vi "Read GPS.vi"(0 "VISA resource name":refnum<visa-resource-name>="COM1", 5 "timeout (ms)":u32=10000, 7 "UTC Time Zone":i32=-5, 9 "stop":bool, 11 "error in (no error)":errorcluster) -> (4 "GPS Data":T1 {"Course over ground (degrees)" format="%#.6g"; "Speed over ground (knots)" format="%#.6g"; "Magnetic Variation (degrees)" format="%#.6g"; "Longitude (ddmm.mmmm)" format="%#.6g"; "Lattitude (ddmm.mmmm)" format="%#.6g"}, 6 "GPS Data Valid?":bool, 10 "Stopped?":bool, 15 "error out":errorcluster)   [LabVIEW 2011]
doc: "This subVI decodes the most common NMEA-0183 sentence transmitted by GPS receivers, the $GPRMC sentence. The subvi returns time, position, ground speed, and magnetic variation. In the GPS interface configuration, use the \"NMEA OUT\" setting and set the baud rate to the standard 4800 bps setting. Connected to the computer's serial port using a PC Interface Cable, available from the GPS vendor. This subvi initializes the serial port on first call. On subsequent calls, the initialization is skipped. Always use the Stop input when stopping the VI so that the serial port connection is closed."
uses:
  <vilib>/Instr/_visa.llb/VISA Configure Serial Port (Instr).vi
panel:
  in  "Cluster":T1 {"Course over ground (degrees)" format="%_4g"; "Speed over ground (knots)" format="%_3g"; "Magnetic Variation (degrees)" format="%_4g"; "Longitude (ddmm.mmmm)" format="%_8g"; "Lattitude (ddmm.mmmm)" format="%_8g"}
  out "Variation East/West":string
  out "Magnetic Variation (degrees)":dbl format="%_4g"
  out "Course over ground (degrees)":dbl format="%_4g"
  out "Speed over ground (knots)":dbl format="%_3g"
  out "Longitude East/West":string
  out "Longitude (ddmm.mmmm)":dbl format="%_8g"
  out "Lattitude North/South":string
  out "Lattitude (ddmm.mmmm)":dbl format="%_8g"
  out "Local Time":timestamp
  out "UTC Time":timestamp
  in  "date time rec":T2
  out "Bytes read":u32
  out "String Read":string="\n"
  # "This subVI decodes the most common NMEA-0183 sentence transmitted by GPS receivers, the $GPRMC sentence. The subvi returns time, position, ground speed, and magnetic variation. In the GPS interface configuration, use the \"NMEA OUT\" setting and set the baud rate to the standard 4800 bps setting. Connected to the computer's serial port using a PC Interface Cable, available from the GPS vendor. This subvi initializes the serial port on first call. On subsequent calls, the initialization is skipped. Always use the Stop input when stopping the VI so that the serial port connection is closed."
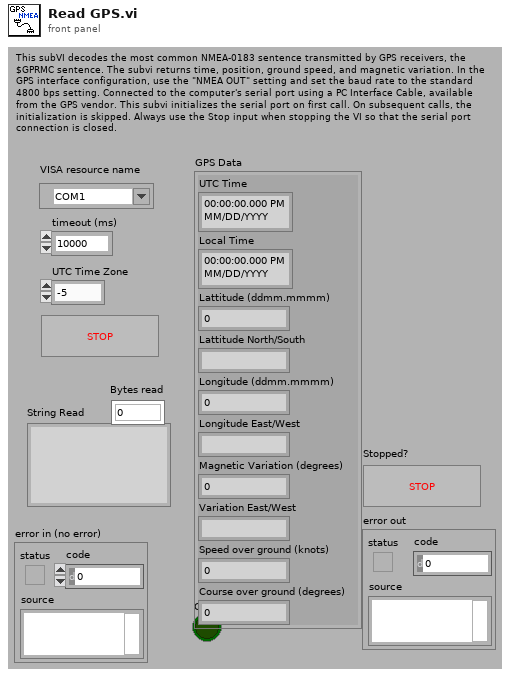
[diagram p1: front panel]
types:
  T1 = cluster{"UTC Time":timestamp, "Local Time":timestamp, "Lattitude (ddmm.mmmm)":dbl, "Lattitude North/South":string, "Longitude (ddmm.mmmm)":dbl, "Longitude East/West":string, "Magnetic Variation (degrees)":dbl, "Variation East/West":string, "Speed over ground (knots)":dbl, "Course over ground (degrees)":dbl}
  T2 = cluster{"second":i32, "minute":i32, "hour":i32, "day of month":i32, "month":i32, "year":i32, "day of week":i32, "day of year":i32, "is DST":i32}
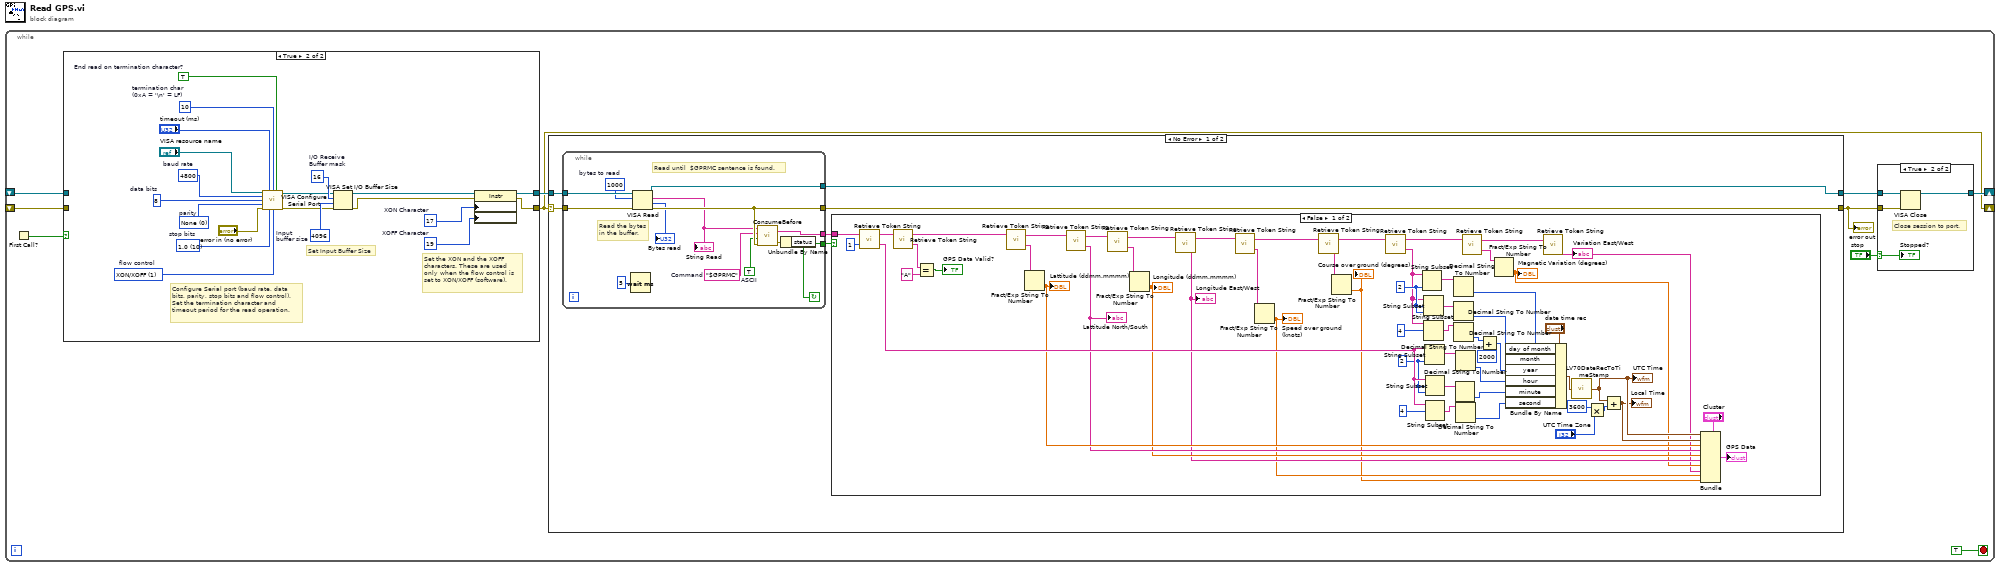
[diagram p0: block diagram]
diagram:
  n1 = while {
    shift-right: [w5] -> _
    shift-left: _ -> [w4]
    shift-right: [w3] -> _
    shift-left: _ -> [w2]
    stop <- TRUE stop-if-true
    n2 = First Call?() -> (First Call?: T/F=w8:bool)
    n3 = case shown="True" w8 {
      tunnel: [w16 w21] -> w10
      tunnel: [w15 w18] -> w3
      tunnel: w4 -> [w16 _]
      tunnel: w2 -> [w15 _]
      frame False {
      }
      frame True {
        w31 = TRUE  # End read on termination character?
        w23 = u8 19  # XOFF Character
        w24 = u8 17  # XON Character
        w29 = u32 4096  # Input buffer size
        w27 = u16 1 items=["None"=0, "XON/XOFF"=1, "RTS/CTS"=2, "DTR/DSR"=4]  # flow control
        w33 = u16 10 items=["1.0"=10, "1.5"=15, "2.0"=20]  # stop bits
        w34 = u16 0 items=["None", "Odd", "Even", "Mark", "Space"]  # parity
        w22 = u16 8  # data bits
        w36 = u32 4800  # baud rate
        w28 = u8 10  # termination char (0xA = '\n' = LF)
        w30 = u16 16  # I/O Receive Buffer mask
        # "Set the XON and the XOFF\ncharacters. These are used\nonly when the flow control is\nset to XON/XOFF (software)."
        # "Configure Serial port (baud rate, data\nbits, parity, stop bits and flow control).\nSet the termination character and\ntimeout period for the read operation."
        # "Set Input Buffer Size"
        n4 = call-poly "VISA Configure Serial Port"("VISA resource name"="VISA resource name", "timeout (10sec)"="timeout (ms)", "termination char\n(0xA = '\\n' = LF)"=w28, "Enable Termination\nChar (T)"=w31, "baud rate (9600)"=w36, "data bits (8)"=w22, "parity (0:none)"=w34, "error in (no error)"="error in (no error)", "stop bits (10: 1 bit)"=w33, "flow control (0:none)"=w27) -> ("VISA resource name out"=w20:refnum<visa-resource-name>, "error out"=w19:errorcluster)  [unwired: 4 in]
        n5 = VISA Set I/O Buffer Size(VISA resource name=w20, mask (16)=w30, size (4096)=w29, error in (no error)=w19) -> (VISA resource name out=w26:refnum<visa-resource-name>, error out=w25:errorcluster)
        n6 = property class="Instr"(reference=w26, error in=w25, "Serial Settings:Flow Control XON Character"=w24, "Serial Settings:Flow Control XOFF Character"=w23) -> (reference out=w21:refnum<visa-resource-name>, error out=w18:errorcluster)
      }
    }
    n7 = case shown="No Error" w3 {
      selector: w3 -> [w39 w113]
      tunnel: w10 -> [w42 w114]
      tunnel: [w41 w114] -> w9
      tunnel: [w40 w113] -> w1
      frame No Error {
        n8 = while {
          tunnel: w42 -> [w55]
          tunnel: [w54] -> w41
          tunnel: [w53] -> w40
          tunnel: w39 -> [w52]
          tunnel: [w48] -> w38
          tunnel: [w44] -> w37
          stop <- w44 continue-if-true
          w46 = u32 1000  # bytes to read
          w51 = "$GPRMC"  # Command
          w50 = TRUE  # ASCII
          # "Read until  $GPRMC sentence is found."
          # "Read the bytes\nin the buffer."
          n9 = Wait (ms)(milliseconds to wait=u32 5 ("millisecond multiple")) -> ()  [unwired: 1 out]
          n10 = VISA Read(VISA resource name=w55, byte count=w46, error in (no error)=w52) -> (VISA resource name out=w54:refnum<visa-resource-name>, read buffer=w49:string, return count=→"Bytes read":u32, error out=w53:errorcluster)
          "String Read" <- w49
          n11 = call <vilib>:"ConsumeBefore.vi"("error in"=w53, "ASCII"=w50, "Before"=w51, "Response String In"=w49) -> ("error out"=w47:errorcluster, "Response String Out"=w48:string)
          n12 = Unbundle By Name(w47) -> ("status"=w44:bool)
        }
        n13 = case shown="False" w37 {
          tunnel: w38 -> [w110 _]
          frame False {
            w78 = 2 ("length (rest)")
            w100 = 2 ("length (rest)")
            n14 = call "Retrieve Token String.vi"("Offset (0)"=1, "input string"=w110) -> ("token string"=w107:string, "output string"=w108:string)
            n15 = call "Retrieve Token String.vi"("input string"=w108) -> ("token string"=w112:string, "output string"=w106:string)  [unwired: 1 in]
            n16 = Equal?(x=w112, y="A") -> (x = y?=→"GPS Data Valid?":bool)
            n17 = call "Retrieve Token String.vi"("input string"=w106) -> ("token string"=w91:string, "output string"=w90:string)  [unwired: 1 in]
            n18 = Fract/Exp String To Number(string=w91) -> (number=w65:dbl)  [unwired: 3 in, 1 out]
            "Lattitude (ddmm.mmmm)" <- w65
            n19 = call "Retrieve Token String.vi"("input string"=w90) -> ("token string"=w64:string, "output string"=w89:string)  [unwired: 1 in]
            "Lattitude North/South" <- w64
            n20 = call "Retrieve Token String.vi"("input string"=w89) -> ("token string"=w88:string, "output string"=w87:string)  [unwired: 1 in]
            n21 = Fract/Exp String To Number(string=w88) -> (number=w63:dbl)  [unwired: 3 in, 1 out]
            "Longitude (ddmm.mmmm)" <- w63
            n22 = call "Retrieve Token String.vi"("input string"=w87) -> ("token string"=w62:string, "output string"=w86:string)  [unwired: 1 in]
            "Longitude East/West" <- w62
            n23 = call "Retrieve Token String.vi"("input string"=w86) -> ("token string"=w85:string, "output string"=w84:string)  [unwired: 1 in]
            n24 = Fract/Exp String To Number(string=w85) -> (number=w59:dbl)  [unwired: 3 in, 1 out]
            "Speed over ground (knots)" <- w59
            n25 = call "Retrieve Token String.vi"("input string"=w84) -> ("token string"=w83:string, "output string"=w82:string)  [unwired: 1 in]
            n26 = Fract/Exp String To Number(string=w83) -> (number=w58:dbl)  [unwired: 3 in, 1 out]
            "Course over ground (degrees)" <- w58
            n27 = call "Retrieve Token String.vi"("input string"=w82) -> ("token string"=w76:string, "output string"=w70:string)  [unwired: 1 in]
            n28 = String Subset(string=w76, length (rest)=w78) -> (substring=w77:string)  [unwired: 1 in]
            n29 = String Subset(string=w76, offset (0)=w78, length (rest)=w78) -> (substring=w79:string)
            n30 = String Subset(string=w76, offset (0)=4) -> (substring=w81:string)  [unwired: 1 in]
            n31 = String Subset(string=w107, length (rest)=w100) -> (substring=w104:string)  [unwired: 1 in]
            n32 = String Subset(string=w107, offset (0)=w100, length (rest)=w100) -> (substring=w98:string)
            n33 = String Subset(string=w107, offset (0)=4) -> (substring=w96:string)  [unwired: 1 in]
            n34 = Decimal String To Number(string=w79) -> (number=w74:i32)  [unwired: 2 in, 1 out]
            n35 = Decimal String To Number(string=w77) -> (number=w75:i32)  [unwired: 2 in, 1 out]
            n36 = Decimal String To Number(string=w81) -> (number=w73:i32)  [unwired: 2 in, 1 out]
            n37 = Decimal String To Number(string=w98) -> (number=w99:i32)  [unwired: 2 in, 1 out]
            n38 = Decimal String To Number(string=w104) -> (number=w101:i32)  [unwired: 2 in, 1 out]
            n39 = Decimal String To Number(string=w96) -> (number=w95:i32)  [unwired: 2 in, 1 out]
            n40 = call "Retrieve Token String.vi"("input string"=w70) -> ("token string"=w69:string, "output string"=w68:string)  [unwired: 1 in]
            n41 = Add(x=w73, y=2000) -> (x+y=w71:i32)
            n42 = Fract/Exp String To Number(string=w69) -> (number=w61:dbl)  [unwired: 3 in, 1 out]
            "Magnetic Variation (degrees)" <- w61
            n43 = Bundle By Name(cluster="date time rec", "day of month"=w75, "month"=w74, "year"=w71, "hour"=w101, "minute"=w99, "second"=w95) -> (w103:T2)
            n44 = call "Retrieve Token String.vi"("input string"=w68) -> ("token string"=w60:string)  [unwired: 1 in, 1 out]
            "Variation East/West" <- w60
            n45 = call <vilib>:"LV70DateRecToTimeStamp.vi"("date time rec"=w103) -> ("Time Stamp"=w67:timestamp)
            "UTC Time" <- w67
            n46 = Multiply(x=3600 ("number"), y="UTC Time Zone") -> (x*y=w92:i32)
            n47 = Add(x=w67, y=w92) -> (x+y=w66:timestamp)
            "Local Time" <- w66
            n48 = Bundle(cluster="Cluster", "UTC Time"=w67, "Local Time"=w66, "Lattitude (ddmm.mmmm)"=w65, "Lattitude North/South"=w64, "Longitude (ddmm.mmmm)"=w63, "Longitude East/West"=w62, "Magnetic Variation (degrees)"=w61, "Variation East/West"=w60, "Speed over ground (knots)"=w59, "Course over ground (degrees)"=w58) -> (→"GPS Data":T1)
          }
          frame True {
          }
        }
      }
      frame Error {
      }
    }
    "error out" <- w1
    n49 = case shown="True" "stop" {
      selector: "stop" -> [_ w12]
      tunnel: w9 -> [w11 w13]
      tunnel: w1 -> [_ w14]
      tunnel: [w11 w13] -> w5
      frame False {
      }
      frame True {
        # "Close session to port."
        n50 = VISA Close(VISA resource name=w13, error in (no error)=w14) -> ()  [unwired: 1 out]
        "Stopped?" <- w12
      }
    }
  }
